vi "Read.vi"(8 "error in (no error)":errorcluster, 11 "Boolean in":refnum<class "Abs_Boolean.lvclass">) -> (0 "error out":errorcluster, 2 "Boolean":bool, 3 "Boolean out":refnum<class "Abs_Boolean.lvclass">)   [LabVIEW 2021, in "Abs_Boolean.lvclass"]
uses:
  Abs_Boolean.lvclass
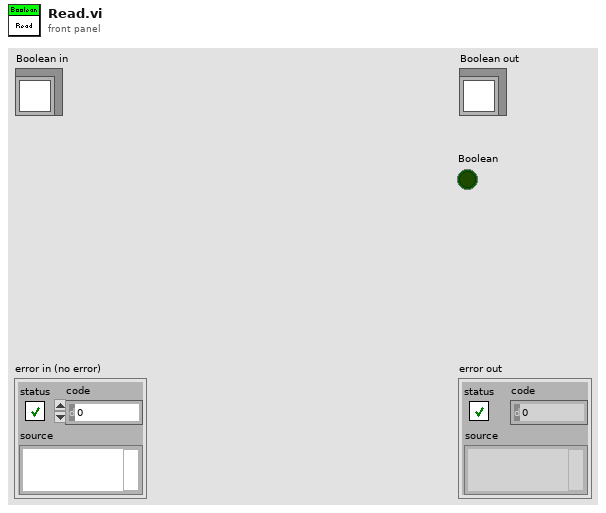
[diagram p1: front panel]
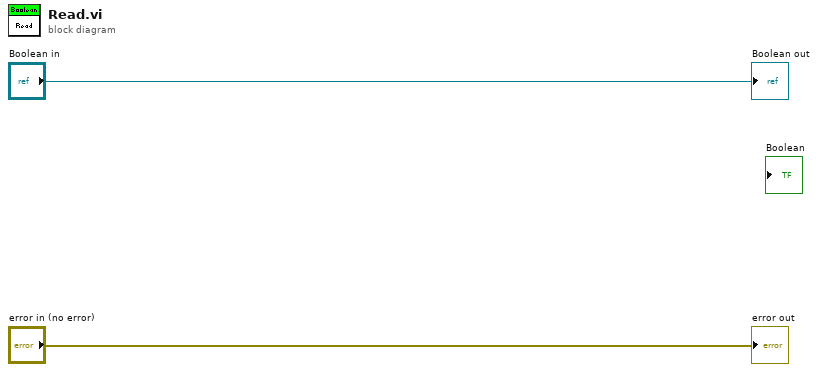
[diagram p0: block diagram]
diagram:
  "error out" <- "error in (no error)"
  "Boolean out" <- "Boolean in"
